vi "Check InitCallback Acknowledgement.vi"(8 "error in (no error)":errorcluster, 11 "InitCallbackAck Registration":refnum<event-registration>) -> (0 "error out":errorcluster)   [LabVIEW 2019]
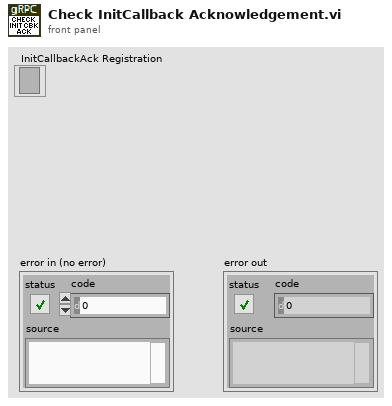
[diagram p1: front panel]
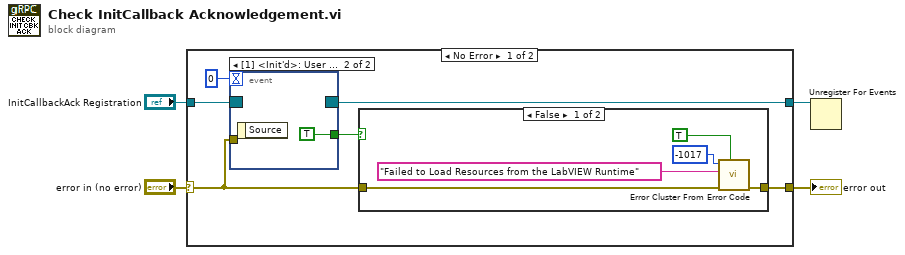
[diagram p0: block diagram]
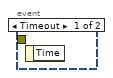
[diagram p3: hidden frame]
diagram:
  n1 = case shown="No Error" "error in (no error)" {
    selector: "error in (no error)" -> [w5 w19]
    tunnel: "InitCallbackAck Registration" -> [w10 w18]
    tunnel: [w9 w18] -> w2
    tunnel: [w8 w19] -> w4
    frame No Error {
      n2 = event shown="[1] <Init'd>: User Event" {
        selector: w10 -> [_ _]
        dyn-events: [_ _] -> w9
        timeout: 0 -> [_ _]
        tunnel: w5 -> [_ _]
        tunnel: [_ TRUE] -> w7
        event Timeout {
          n3 = event-data() -> ()  [unwired: 1 in, 1 out]
        }
        event User Event {
          n4 = event-data() -> ()  [unwired: 1 in, 1 out]
        }
      }
      n5 = case shown="False" w7 {
        tunnel: w5 -> [w12 w16]
        tunnel: [w11 w16] -> w8
        frame False {
          n6 = call <vilib>:"Error Cluster From Error Code.vi"("show call chain? (False)"=TRUE, "error in (no error)"=w12, "error message (\"\")"="Failed to Load Resources from the LabVIEW Runtime" ("error message (\"\")"), "error code (0)"=-1017) -> ("error out"=w11:errorcluster)  [unwired: 5 in]
        }
        frame True {
        }
      }
    }
    frame Error {
    }
  }
  "error out" <- w4
  n7 = Unregister For Events(event registration refnum=w2) -> ()  [unwired: 1 in, 1 out]
